vi "Rosser Matrix (DBL).vi"() -> (3 "Rosser Matrix":T1)   [LabVIEW 2014, in "NI_AALPro.lvlib"]
uses:
  NI_AALPro.lvlib
  RealMatrix.ctl
  NI_Matrix.lvlib
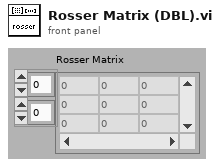
[diagram p1: front panel]
types:
  T1 = typedef "NI_Matrix.lvlib/RealMatrix.ctl" = dbl[][]
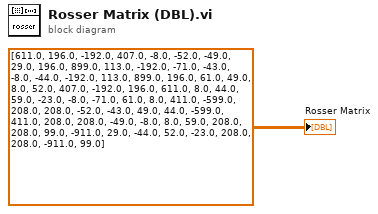
[diagram p0: block diagram]
diagram:
  "Rosser Matrix" <- dbl[][] [[611.0, 196.0, -192.0, 407.0, -8.0, -52.0, -49.0, 29.0], [196.0, 899.0, 113.0, -192.0, -71.0, -43.0, -8.0, -44.0], [-192.0, 113.0, 899.0, 196.0, 61.0, 49.0, 8.0, 52.0], [407.0, -192.0, 196.0, 611.0, 8.0, 44.0, 59.0, -23.0], [-8.0, -71.0, 61.0, 8.0, 411.0, -599.0, 208.0, 208.0], [-52.0, -43.0, 49.0, 44.0, -599.0, 411.0, 208.0, 208.0], [-49.0, -8.0, 8.0, 59.0, 208.0, 208.0, 99.0, -911.0], [29.0, -44.0, 52.0, -23.0, 208.0, 208.0, -911.0, 99.0]] ("rosser")
